vi "Set Title Text Color.vi"(8 "error in (no error)":errorcluster, 10 "Color Box":u32(colorbox)) -> (0 "error out":errorcluster)   [LabVIEW 2013, in "Progress Bar.lvlib"]
uses:
  Progress Bar.lvlib
  Queue/Queue Action.ctl
  Queue/Property Message.ctl
  Queue/Property Action.ctl
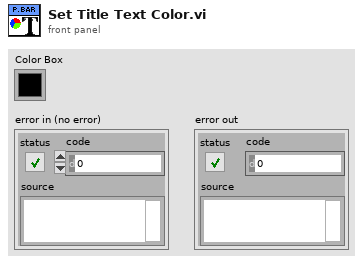
[diagram p1: front panel]
types:
  T1 = typedef "Progress Bar.lvlib/Property Message.ctl" = cluster{"Property":T2, "Value":variant}
  T2 = typedef "Progress Bar.lvlib/Property Action.ctl" = enum16{"BG Color", "Timeout", "Title Text Color", "Title Text", "Action Text Color", "Action Text", "Bar Color", "Set Slider Value", "Add to Slider Value", "Exit"}
  T3 = typedef "Progress Bar.lvlib/Queue Action.ctl" = enum16{"Obtain Queue", "Release Queue", "Get Queue"}
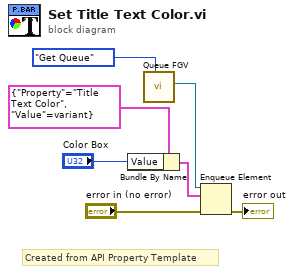
[diagram p0: block diagram]
diagram:
  # "Created from API Property Template"
  n1 = Bundle By Name(cluster=T1 {"Property"=enum."Title Text Color", "Value"=variant} ("element"), "Value"="Color Box") -> (w3:T1)
  n2 = call "Queue FGV.vi"("Enum"=Queue_Action."Get Queue") -> ("queue out"=w6:refnum<queue>)  [unwired: 9 in, 1 out]
  n3 = Enqueue Element(queue=w6, element=w3, error in (no error)="error in (no error)") -> (error out=→"error out":errorcluster)  [unwired: 1 in, 2 out]
